vi "VisionAngle.vi"(1 "XPos":dbl(slide) scale=0.0..640.0, 2 "ImageWidth":dbl, 3 "ViewAngle":dbl) -> (0 "AngleOfDeviation":dbl)   [LabVIEW 2016]
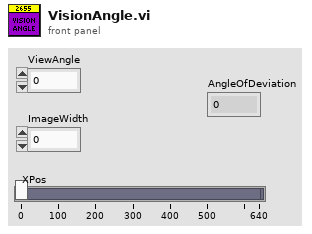
[diagram p1: front panel]
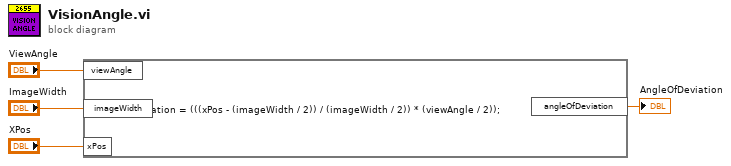
[diagram p0: block diagram]
diagram:
  n1 = formula code="angleOfDeviation = (((xPos - (imageWidth / 2)) / (imageWidth / 2)) * (viewAngle / 2));"("viewAngle"="ViewAngle", "imageWidth"="ImageWidth", "xPos"="XPos") -> ("angleOfDeviation"=→"AngleOfDeviation":dbl)
